vi "killProcess.vi"(8 "error in (no error)":errorcluster, 10 "pathOfProcess":path, 11 "SalProcess in":refnum<class "SalProcess.lvclass">) -> (0 "error out":errorcluster, 2 "isRemoved":bool, 3 "SalProcess out":refnum<class "SalProcess.lvclass">)   [LabVIEW 2018, in "SalProcess.lvclass"]
doc: "Kill the process that is running in the background."
uses:
  SalProcess.lvclass
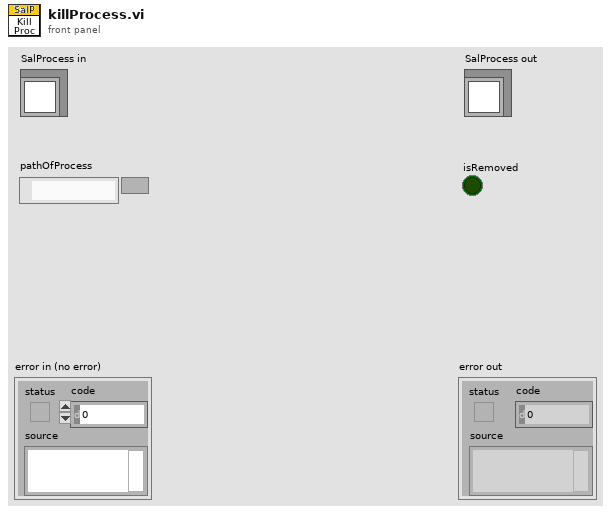
[diagram p1: front panel]
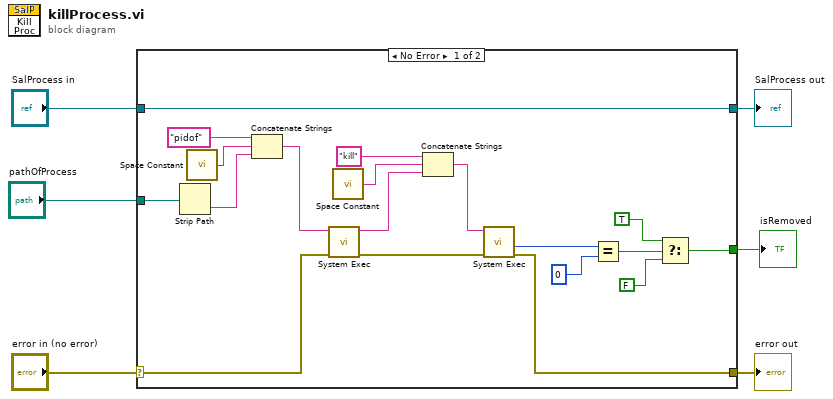
[diagram p0: block diagram]
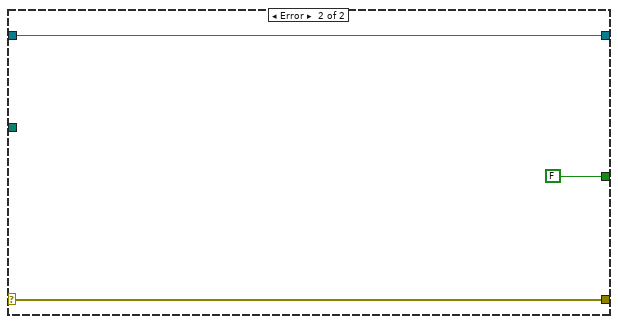
[diagram p2: hidden frame]
diagram:
  n1 = case shown="No Error" "error in (no error)" {
    selector: "error in (no error)" -> [w19 w28]
    tunnel: [w13 w28] -> w5
    tunnel: [w25 w27] -> w3
    tunnel: "SalProcess in" -> [w25 w27]
    tunnel: "pathOfProcess" -> [w24 _]
    tunnel: [w7 FALSE] -> w1
    frame No Error {
      n2 = Strip Path(path=w24) -> (name=w21:string)  [unwired: 1 out]
      n3 = call <vilib>:"Space Constant.vi"() -> ("String"=w22:string)
      n4 = Concatenate Strings("pidof", w22, w21) -> (w20:string)
      n5 = call <vilib>:"System Exec.vi"("error in (no error)"=w19, "command line"=w20) -> ("error out"=w15:errorcluster, "standard output"=w16:string)  [unwired: 6 in, 2 out]
      n6 = call <vilib>:"Space Constant.vi"() -> ("String"=w17:string)
      n7 = Concatenate Strings("kill", w17, w16) -> (w14:string)
      n8 = call <vilib>:"System Exec.vi"("error in (no error)"=w15, "command line"=w14) -> ("error out"=w13:errorcluster, "return code"=w12:i32)  [unwired: 6 in, 2 out]
      n9 = Equal?(x=w12, y=0) -> (x = y?=w10:bool)
      n10 = Select(t=TRUE, s=w10, f=FALSE) -> (s? t:f=w7:bool)
    }
    frame Error {
    }
  }
  "error out" <- w5
  "SalProcess out" <- w3
  "isRemoved" <- w1
